vi "cRIO_FPGA_COMMUNICATION Lese Eingangsdaten.vi"(8 "error in (no error)":errorcluster caption="Fehler (Eingang, kein Fehler)", 11 "Station Index":T1) -> (0 "error out":errorcluster caption="Fehler (Ausgang)", 2 "Station":bool[](array[boolean]), 3 "Band":bool[](array[boolean]))   [LabVIEW 2013, in "cRIO_FPGA_COMMUNICATION.lvlib"]
uses:
  cRIO_FPGA_COMMUNICATION.lvlib
  TYPES/TYPE Station Index.ctl
  TYPES/TYPE Band und Stations Kommandos.ctl
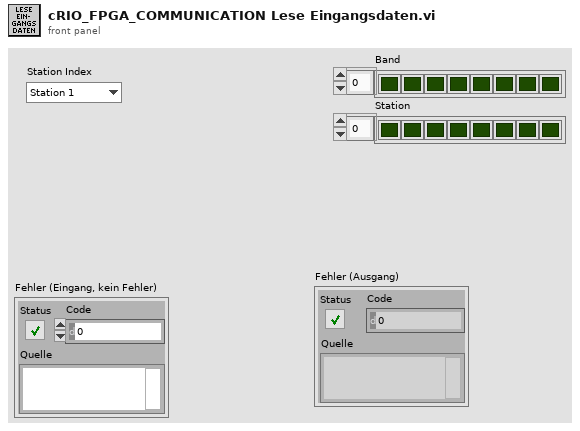
[diagram p1: front panel]
types:
  T1 = typedef "cRIO_FPGA_COMMUNICATION.lvlib/TYPE Station Index.ctl" = enum16{"Station 1", "Station 2", "Station 3", "Station 4", "Station 5", "Station 6", "Station 7", "Station 8", "Station 9", "Station 10", "Station 11", "Station 12", "Station 13", "Station 14", "Station 15", "Station 16", "Station 17", "Station 18", "Station 19", "Station 20"}
  T2 = typedef "cRIO_FPGA_COMMUNICATION.lvlib/TYPE Band und Stations Kommandos.ctl" = enum16{"Init", "Lese", "Schreibe"}
  T3 = typedef "cRIO_FPGA_COMMUNICATION.lvlib/TYPE Band Lese Daten.ctl" = cluster{"Band":bool[], "Station":bool[], "Band Zähler":i32, "Letzter Bandzählerwert":bool}
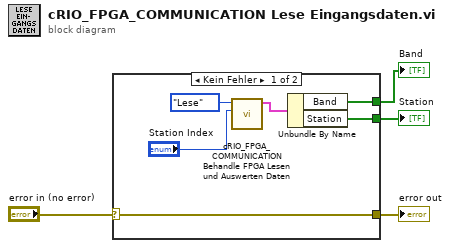
[diagram p0: block diagram]
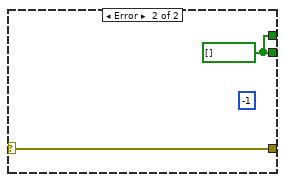
[diagram p2: hidden frame]
diagram:
  n1 = case shown="Kein Fehler" "error in (no error)" {
    selector: "error in (no error)" -> [w10 w12]
    tunnel: [w10 w12] -> w3
    tunnel: [w6 w11] -> w2
    tunnel: [w5 w11] -> w1
    frame No Error {
      n2 = call "cRIO_FPGA_COMMUNICATION Behandle FPGA Lesen und Auswerten Daten.vi"("Station Index"="Station Index", "FGV Band/Station Commands"=TYPE_Band_und_Stations_Kommandos."Lese") -> ("Band/Station Lese Daten"=w7:T3)  [unwired: 9 in]
      n3 = Unbundle By Name(w7) -> ("Band"=w6:bool[], "Station"=w5:bool[])
    }
    frame Error {
      (unwired) -1 ("Band Zähler")
      w11 = bool[] [] ("Band")
    }
  }
  "error out" <- w3
  "Band" <- w2
  "Station" <- w1
